vi "StateBallHandling.vi"(0 "Master State In":enum16{"Speaker", "Amp", "Climbing", "Trap"}(ring)=enum."Trap") -> ()   [LabVIEW 2023]
doc: "This VI performs all of the calculations and decisions related to the swerve drive."
uses:
  GlobalDriverStationCommands.vi
  GlobalBallHandling.vi
panel:
  in  "Shooter Rotating":bool
  in  "Force Shoot":bool
  in  "Indexer Shooter Power":dbl=0.2
  in  "Spun up":bool
  in  "Shooting":bool
  in  "Intake Threshold":u32=300
  in  "Force Intake":bool
  in  "Elevator down":bool
  in  "Indexer Power":dbl=0.2
  in  "Rotator Power":dbl=0.1
  in  "Intake Power":dbl=0.5
  in  "Intaking":bool
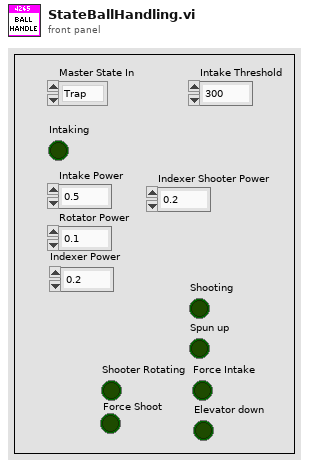
[diagram p1: front panel]
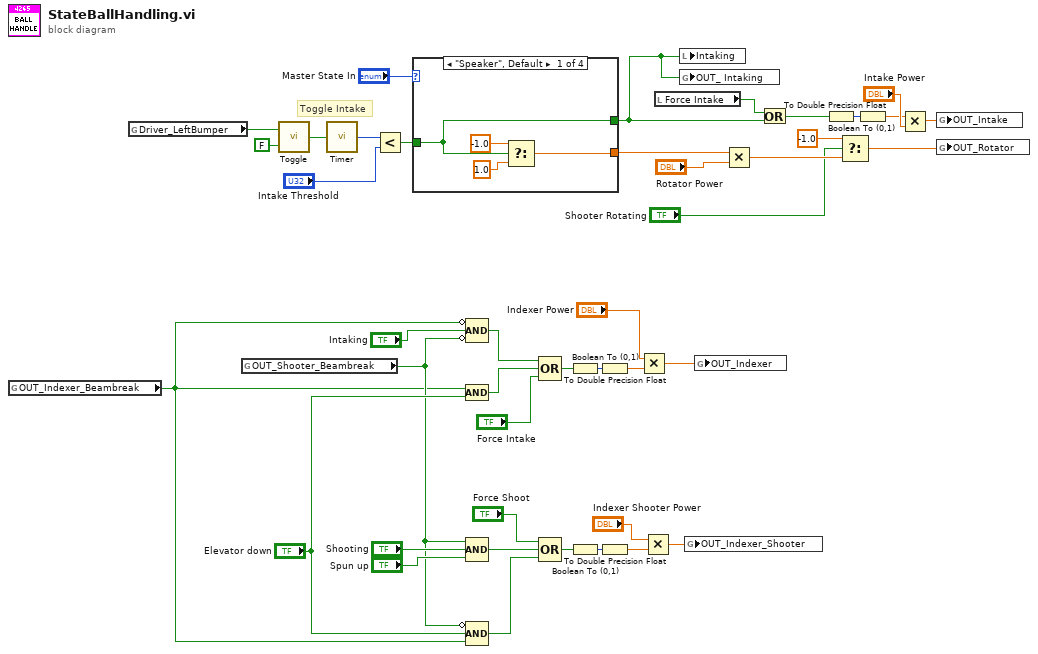
[diagram p0: block diagram]
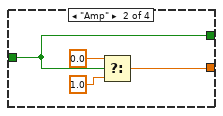
[diagram p2: hidden frame]
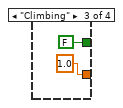
[diagram p3: hidden frame]
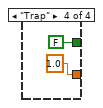
[diagram p4: hidden frame]
diagram:
  # "Toggle Intake"
  n1 = global read "GlobalBallHandling.vi" "OUT_Indexer_Beambreak"() -> (w5:bool)
  n2 = global read "GlobalDriverStationCommands.vi" "Driver_LeftBumper"() -> (w42:bool)
  n3 = global read "GlobalBallHandling.vi" "OUT_Shooter_Beambreak"() -> (w6:bool)
  n4 = call "Toggle.vi"("Initial State"=FALSE, "Trigger"=w42) -> ("New State"=w27:bool)
  n5 = call "Timer.vi"("Reset Timer"=w27) -> ("Time (ms)"=w26:u32)
  n6 = Less?(x=w26, y="Intake Threshold") -> (x < y?=w12:bool)
  n7 = case shown="\"Speaker\", Default" "Master State In" {
    tunnel: w12 -> [w43 w48 _ _]
    tunnel: [w46 w49 1.0 ("t") 1.0 ("t")] -> w39
    tunnel: [w43 w48 FALSE FALSE] -> w7
    frame "Speaker", Default {
      n8 = Select(t=-1.0, s=w43, f=1.0 ("t")) -> (s? t:f=w46:dbl)
    }
    frame "Amp" {
      n9 = Select(t=0.0, s=w48, f=1.0 ("t")) -> (s? t:f=w49:dbl)
    }
    frame "Climbing" {
    }
    frame "Trap" {
    }
  }
  n10 = Compound Arithmetic op=AND(invert w5, "Intaking", invert w6) -> (w30:bool)
  n11 = Compound Arithmetic op=AND(w5, "Elevator down") -> (w29:bool)
  n12 = Compound Arithmetic op=AND(w6, "Shooting", "Spun up") -> (w18:bool)
  n13 = Compound Arithmetic op=AND(invert w6, "Elevator down", w5) -> (w17:bool)
  n14 = Compound Arithmetic op=OR(w30, w29, "Force Intake") -> (w28:bool)
  n15 = Compound Arithmetic op=OR("Force Shoot", w18, w17) -> (w19:bool)
  n16 = Boolean To (0,1)(Boolean=w28) -> (0, 1=w38:i16)
  n17 = Boolean To (0,1)(Boolean=w19) -> (0, 1=w24:i16)
  n18 = To Double Precision Float(number=w38) -> (double precision float=w37:dbl)
  n19 = To Double Precision Float(number=w24) -> (double precision float=w23:dbl)
  n20 = Multiply(x="Indexer Power", y=w37) -> (x*y=w35:dbl)
  n21 = Multiply(x="Indexer Shooter Power", y=w23) -> (x*y=w15:dbl)
  n22 = local read "Force Intake"() -> (w8:bool)
  n23 = local write "Intaking"(w7) -> ()
  n24 = global write "GlobalBallHandling.vi" "OUT_ Intaking"(w7) -> ()
  n25 = global write "GlobalBallHandling.vi" "OUT_Indexer_Shooter"(w15) -> ()
  n26 = global write "GlobalBallHandling.vi" "OUT_Indexer"(w35) -> ()
  n27 = Multiply(x=w39, y="Rotator Power") -> (x*y=w4:dbl)
  n28 = Or(x=w8, y=w7) -> (x .or. y?=w9:bool)
  n29 = Boolean To (0,1)(Boolean=w9) -> (0, 1=w10:i16)
  n30 = Select(t=-1.0, s="Shooter Rotating", f=w4) -> (s? t:f=w1:dbl)
  n31 = To Double Precision Float(number=w10) -> (double precision float=w11:dbl)
  n32 = Multiply(x=w11, y="Intake Power") -> (x*y=w36:dbl)
  n33 = global write "GlobalBallHandling.vi" "OUT_Intake"(w36) -> ()
  n34 = global write "GlobalBallHandling.vi" "OUT_Rotator"(w1) -> ()
